vi "FeedbackDecode_UpdateSelPresets.vi"(2 "OldSelIn":bool[](array[boolean]), 3 "NewSelIn":bool[](array[boolean])) -> (0 "OldSelOut":bool[](array[boolean]), 1 "NewSelOut":bool[](array[boolean]))   [LabVIEW 2020]
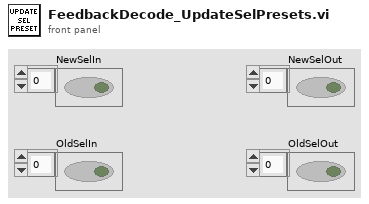
[diagram p1: front panel]
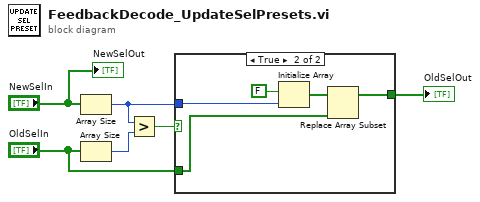
[diagram p0: block diagram]
diagram:
  n1 = Array Size(array="NewSelIn") -> (size(s)=w4:i32)
  n2 = Array Size(array="OldSelIn") -> (size(s)=w6:i32)
  n3 = Greater?(x=w4, y=w6) -> (0:w5:bool)
  n4 = case shown="True" w5 {
    tunnel: w4 -> [_ w10]
    tunnel: "OldSelIn" -> [w7 w9]
    tunnel: [w7 w8] -> w2
    frame False {
    }
    frame True {
      n5 = Initialize Array(FALSE ("new element/subarray"), w10) -> (w12:bool[])
      n6 = Replace Array Subset(array=w12, new element=w9) -> (w8:bool[])  [unwired: 1 in]
    }
  }
  "OldSelOut" <- w2
  "NewSelOut" <- "NewSelIn"
